vi "Train Magnet.vi"(8 "error in (no error)":errorcluster, 11 "Power Supply in":refnum<class "Power Supply.lvclass">) -> (0 "error out":errorcluster, 3 "Power Supply out":refnum<class "Power Supply.lvclass">)   [LabVIEW 2009, in "Power Supply.lvclass"]
uses:
  Power Supply.lvclass
  Power Supply.lvclass/Power Supply.ctl
  Global/Relative Sound Files.vi
panel:
  in  "Training Field and Speed Cluster":T1={"Training Field"=[0.0, 4.108, 5.78], "Training Speed"=[0.0057, 0.0022833333333333334, 0.0011333333333333334]}
  out "active":bool
  out "rate":dbl[unit] caption="Rate"
  in  "interrupt":bool
  out "Original Field":dbl[unit]
  in  "endprogram":bool
  in  "go":bool
  in  "upanddown":bool=TRUE
  in  "Target Field":dbl[unit]
  # "To what field would you like to train the magnet?"
  # "Training means going up to the desired field at the \"train speed\"\nand then coming back down to the starting field, again, at the \"train speed.\" Going to 7 T takes about 42 min, one way."
  # "The speed at index n corresponds to the speed\nfrom field[n] to field[n+1]."
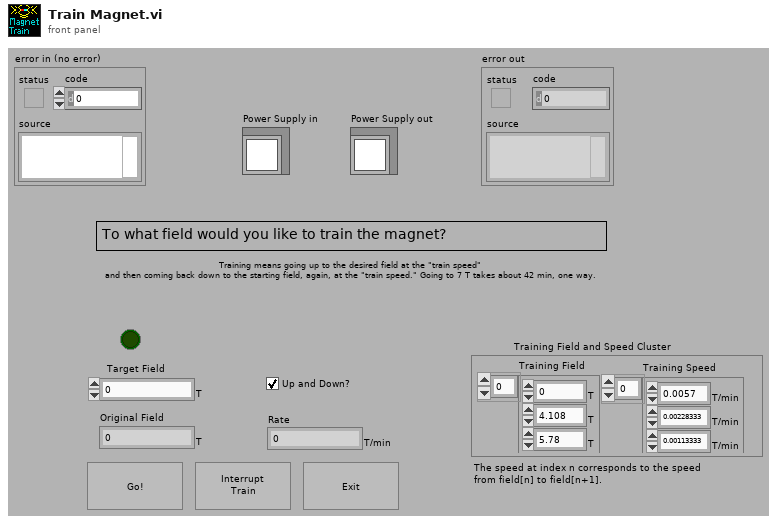
[diagram p1: front panel]
types:
  T1 = cluster{"Training Field":dbl[unit][], "Training Speed":dbl[unit][]}
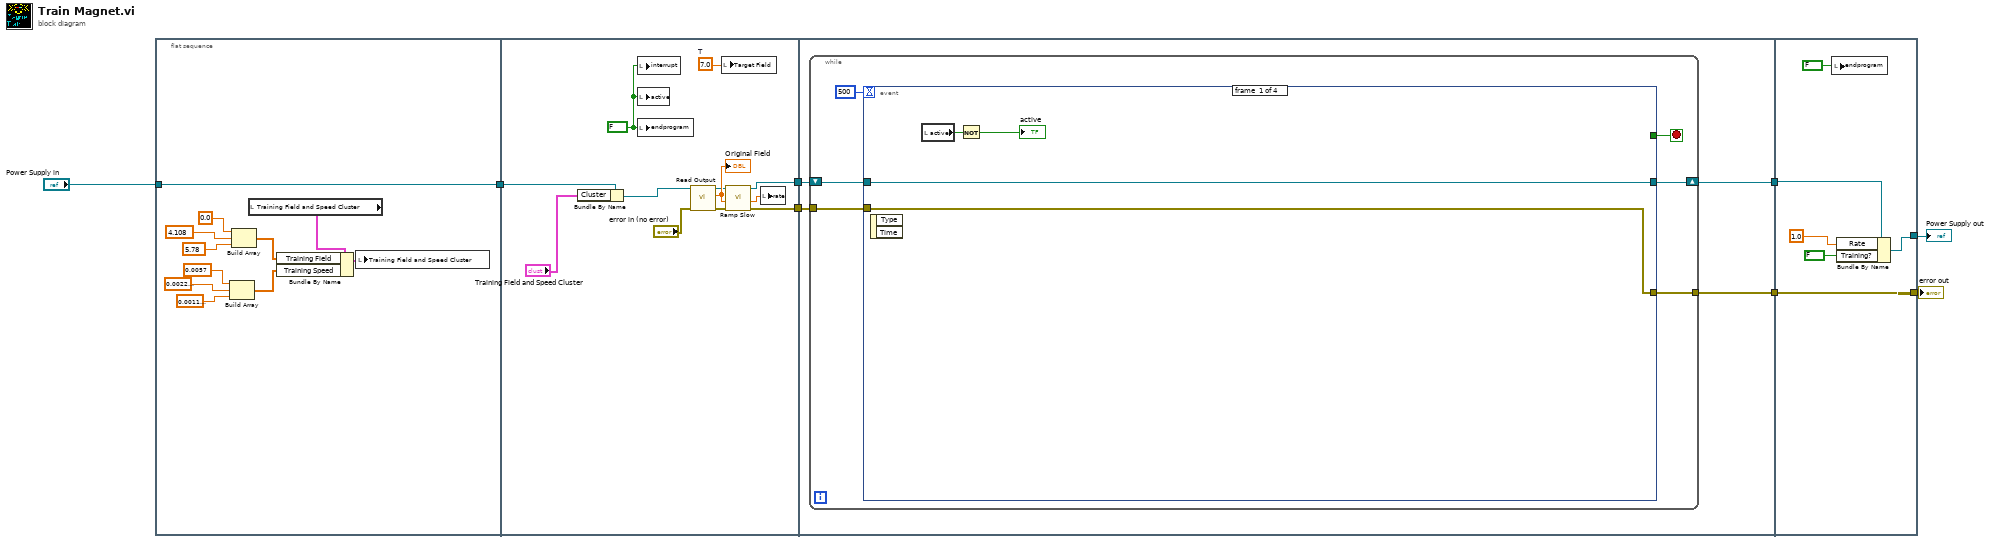
[diagram p0: block diagram]
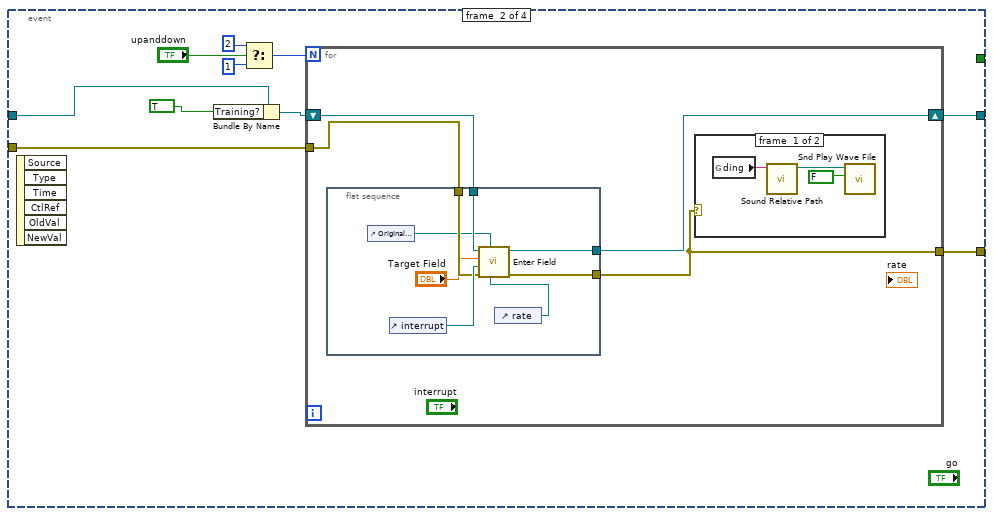
[diagram p2: hidden frame]
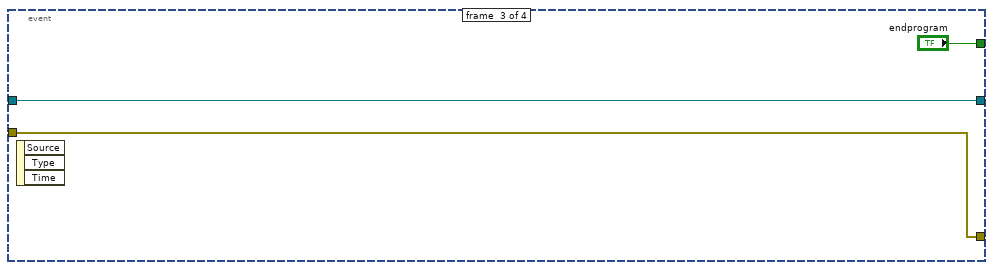
[diagram p4: hidden frame]
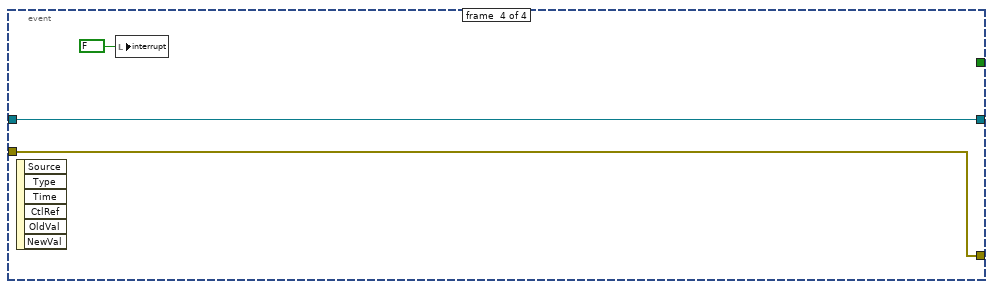
[diagram p5: hidden frame]
diagram:
  n1 = flat-sequence {
    tunnel: "Power Supply in" -> [w19]
    tunnel: [w19] -> w1
    tunnel: [w23] -> w7
    tunnel: [w25] -> w6
    tunnel: w1 -> [w22]
    tunnel: w7 -> [w35]
    tunnel: w6 -> [w34]
    tunnel: [w33] -> w5
    tunnel: [w32] -> w3
    tunnel: w5 -> [w79]
    tunnel: [w78] -> w4
    tunnel: w3 -> [w81]
    tunnel: [w81] -> w2
    frame #0 {
      n2 = Build Array(dbl[unit] 0.0057 ("element"), dbl[unit] 0.0022833333333333334 ("element"), dbl[unit] 0.0011333333333333334 ("element")) -> (w10:dbl[unit][])
      n3 = Build Array(dbl[unit] 0.0 ("element"), dbl[unit] 4.108 ("element"), dbl[unit] 5.78 ("element")) -> (w9:dbl[unit][])
      n4 = local read "Training Field and Speed Cluster"() -> (w18:T1)
      n5 = Bundle By Name(cluster=w18, "Training Field"=w9, "Training Speed"=w10) -> (w17:T1)
      n6 = local write "Training Field and Speed Cluster"(w17) -> ()
    }
    frame #1 {
      w29 = dbl[unit] 7.0  # T
      w30 = FALSE
      n7 = Bundle By Name(cluster=w22, "Cluster"="Training Field and Speed Cluster") -> (w21:refnum<class "Power Supply.lvclass">)
      n8 = local write "interrupt"(w30) -> ()
      n9 = local write "active"(w30) -> ()
      n10 = local write "endprogram"(w30) -> ()
      n11 = call-dynamic "Read Output.vi"("error in (no error)"="error in (no error)", "Power Supply in"=w21) -> ("error out"=w26:errorcluster, "Field"=w28:dbl[unit], "Power Supply out"=w24:refnum<class "Power Supply.lvclass">)  [unwired: 6 in, 1 out]
      "Original Field" <- w28
      n12 = local write "Target Field"(w29) -> ()
      n13 = call-dynamic "Ramp Slow.vi"("error in (no error)"=w26, "fieldIN"=w28, "Power Supply in"=w24) -> ("error out"=w25:errorcluster, "Rate Out"=w31:dbl[unit], "Power Supply out"=w23:refnum<class "Power Supply.lvclass">)  [unwired: 6 in]
      n14 = local write "rate"(w31) -> ()
    }
    frame #2 {
      n15 = while {
        tunnel: [w37] -> w32
        tunnel: w34 -> [w36]
        shift-right: [w38] -> w33
        shift-left: w35 -> [w39]
        stop <- w41 stop-if-true
        n16 = event shown="[1] \"go\": Value Change" {
          selector: _ -> [_ _ _ _]
          dyn-events: _ -> [_ _ _ _]
          timeout: 500 -> [_ _ _ _]
          tunnel: [_ _ "endprogram" _] -> w41
          tunnel: w39 -> [w45 w48 w72 w75]
          tunnel: [w45 w51 w72 w75] -> w38
          tunnel: [w44 w50 w71 w74] -> w37
          tunnel: w36 -> [w44 w49 w71 w74]
          event #0 {
            n17 = event-data() -> ()  [unwired: 3 out]
            n18 = local read "active"() -> (w43:bool)
            n19 = Not(x=w43) -> (.not. x?=→"active":bool)
          }
          event #1 {
            n20 = event-data() -> ()  [unwired: 7 out]
            n21 = Bundle By Name(cluster=w48, "Training?"=TRUE) -> (w47:refnum<class "Power Supply.lvclass">)
            n22 = Select(t=2, s="upanddown", f=1) -> (s? t:f=w52:i32)
            n23 = for {
              N: w52 -> [_]
              shift-right: [w58] -> w51
              shift-left: w47 -> [w59]
              tunnel: [w57] -> w50
              tunnel: w49 -> [w56]
              n24 = flat-sequence {
                tunnel: [w66] -> w57
                tunnel: w59 -> [w65]
                tunnel: [w64] -> w58
                tunnel: w56 -> [w63]
                frame #0 {
                  n25 = control-ref of="Original Field"() -> (w61:refnum<vi>)
                  n26 = control-ref of="interrupt"() -> (w67:refnum<vi>)
                  n27 = control-ref of="rate"() -> (w60:refnum<vi>)
                  n28 = call-dynamic "Enter Field.vi"("rate monitor"=w60, "Field monitor"=w61, "error in (no error)"=w63, "Abort button"=w67, "Target field"="Target Field", "Power Supply in"=w65) -> ("error out"=w66:errorcluster, "Power Supply out"=w64:refnum<class "Power Supply.lvclass">)  [unwired: 4 in]
                }
              }
              n29 = case shown="No Error" w57 {
                frame #0 {
                  n30 = global read "Relative Sound Files.vi" "ding"() -> (w69:string)
                  n31 = call "Sound Relative Path.vi"("Sound"=w69) -> ("Relative Path"=w68:path)  [unwired: 10 in]
                  n32 = call <vilib>:"Snd Play Wave File.vi"("wait until finish (T)"=FALSE, "wave file path"=w68) -> ()  [unwired: 1 in, 9 out]
                }
                frame #1 {
                }
              }
            }
          }
          event #2 {
            n33 = event-data() -> ()  [unwired: 4 out]
          }
          event #3 {
            n34 = event-data() -> ()  [unwired: 7 out]
            n35 = local write "interrupt"(FALSE) -> ()
          }
        }
      }
    }
    frame #3 {
      n36 = local write "endprogram"(FALSE) -> ()
      n37 = Bundle By Name(cluster=w79, "Rate"=dbl[unit] 1.0, "Training?"=FALSE) -> (w78:refnum<class "Power Supply.lvclass">)
    }
  }
  "Power Supply out" <- w4
  "error out" <- w2
